vi "Cleanup.vi"(8 "error in (no error)":errorcluster, 11 "Chat Client in":refnum<class "Chat Client.lvclass">) -> (0 "error out":errorcluster)   [LabVIEW 2020, in "Chat Client.lvclass"]
uses:
  Chat Client.lvclass
  Stream-TCP/TCP Client/TCP Client.lvclass
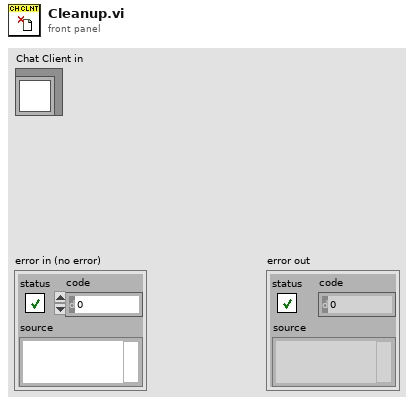
[diagram p1: front panel]
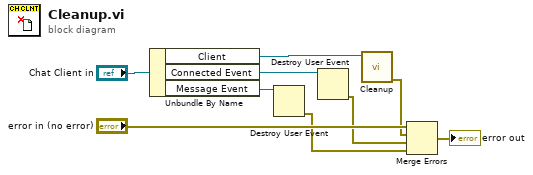
[diagram p0: block diagram]
diagram:
  n1 = Unbundle By Name("Chat Client in") -> ("Client"=w5:refnum<class "TCP Client.lvclass">, "Connected Event"=w6:refnum<user-event>, "Message Event"=w7:refnum<user-event>)
  n2 = Destroy User Event(user event=w7) -> (error out=w1:errorcluster)  [unwired: 1 in]
  n3 = Destroy User Event(user event=w6) -> (error out=w2:errorcluster)  [unwired: 1 in]
  n4 = call-dynamic "Cleanup.vi"("TCP Client in"=w5) -> ("error out"=w3:errorcluster)  [unwired: 10 in]
  n5 = Merge Errors("error in (no error)", w3, w2, w1) -> (→"error out":errorcluster)
